vi "Configure Modulation (Frequency).vi"(0 "VISA resource name":refnum<visa-resource-name>, 1 "Enable Frequency Modulation (T: Enable)":bool=TRUE, 5 "Channel (0: Channel 1)":T1 items=["Channel 1", "Channel 2"], 7 "FM Source (0: Internal)":u16(ring) items=["Internal", "External"], 9 "Modulation Waveform (0: Sine)":u16(ring) items=["Sine", "Square", "Triangle", "Ramp", "Down Ramp", "Noise", "User 1", "User 2", "User 3", "User 4", "EMEMory", "EFILe"], 11 "error in (no error)":errorcluster, 12 "Modulation Frequency (100.00 Hz)":dbl[unit]=100.0, 13 "Peak Deviation (100.00 Hz)":dbl[unit]=100.0) -> (4 "VISA resource name out":refnum<visa-resource-name>, 15 "error out":errorcluster)   [LabVIEW 2009, in "Tektronix AFG 3000 Series.lvlib"]
doc: "Configures and enables frequency modulation (FM). In FM, the frequency of the carrier is varied by the frequency of the modulating waveform."
uses:
  Tektronix AFG 3000 Series.lvlib
  controls.llb/Channel.ctl
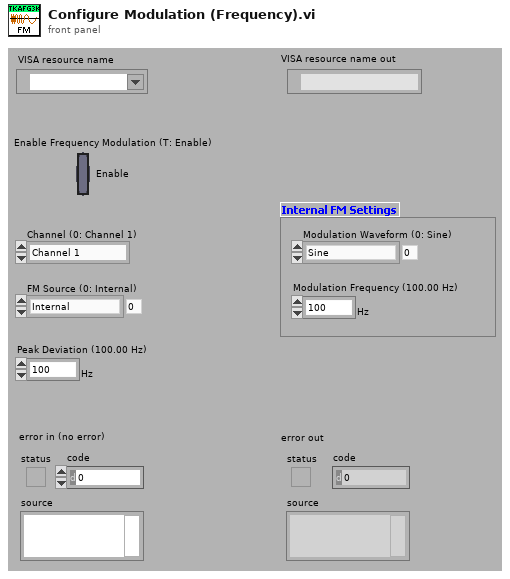
[diagram p1: front panel]
types:
  T1 = typedef "Channel.ctl" = u16
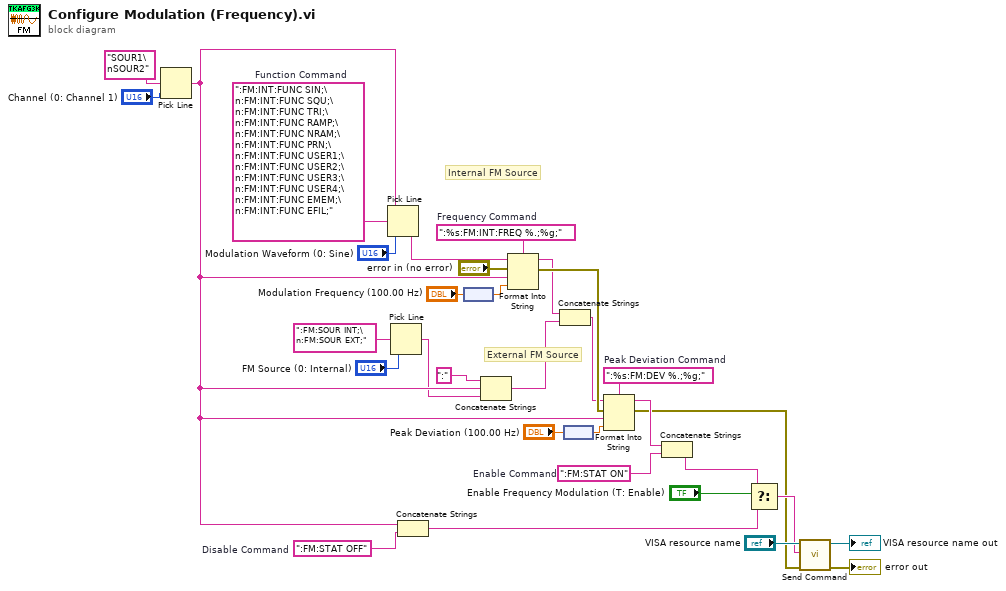
[diagram p0: block diagram]
diagram:
  w19 = ":FM:INT:FUNC SIN;\n:FM:INT:FUNC SQU;\n:FM:INT:FUNC TRI;\n:FM:INT:FUNC RAMP;\n:FM:INT:FUNC NRAM;\n:FM:INT:FUNC PRN;\n:FM:INT:FUNC USER1;\n:FM:INT:FUNC USER2;\n:FM:INT:FUNC USER3;\n:FM:INT:FUNC USER4;\n:FM:INT:FUNC EMEM;\n:FM:INT:FUNC EFIL;"  # Function Command
  w21 = ":%s:FM:INT:FREQ %.;%g;"  # Frequency Command
  w27 = ":FM:STAT ON"  # Enable Command
  w32 = ":%s:FM:DEV %.;%g;"  # Peak Deviation Command
  w24 = ":FM:STAT OFF"  # Disable Command
  # "Internal FM Source"
  # "External FM Source"
  n1 = Pick Line(multi-line string="SOUR1\nSOUR2" ("string (\"\")"), line index="Channel (0: Channel 1)") -> (output string=w5:string)  [unwired: 1 out]
  n2 = Pick Line(string ("")=w5, multi-line string=w19, line index="Modulation Waveform (0: Sine)") -> (output string=w20:string)
  n3 = Pick Line(multi-line string=":FM:SOUR INT;\n:FM:SOUR EXT;" ("Source Command"), line index="FM Source (0: Internal)") -> (output string=w4:string)  [unwired: 1 out]
  n4 = Concatenate Strings(w5, w24) -> (w22:string)
  n5 = node("Modulation Frequency (100.00 Hz)") -> (w14:dbl)
  n6 = Concatenate Strings(":" ("string"), w5, w4) -> (w2:string)
  n7 = Format Into String(format string=w21, initial string=w20, error in="error in (no error)", w5, w14) -> (resulting string=w3:string, error out=w16:errorcluster)
  n8 = Concatenate Strings(w3, w2) -> (w1:string)
  n9 = node("Peak Deviation (100.00 Hz)") -> (w13:dbl)
  n10 = Format Into String(format string=w32, initial string=w1, error in=w16, w5, w13) -> (resulting string=w28:string, error out=w7:errorcluster)
  n11 = Concatenate Strings(w28, w27) -> (w18:string)
  n12 = Select(t=w18, s="Enable Frequency Modulation (T: Enable)", f=w22) -> (s? t:f=w8:string)
  n13 = call "Send Command.vi"("error in (no error)"=w7, "write buffer"=w8, "VISA resource name"="VISA resource name") -> ("error out"=→"error out":errorcluster, "VISA resource name out"=→"VISA resource name out":refnum<visa-resource-name>)  [unwired: 7 out]
